vi "DockerTools - Get container list.vi"(8 "error in":errorcluster) -> (0 "error out":errorcluster, 2 "Container list":string[][](array[string]), 3 "Standard output":string)   [LabVIEW 2017]
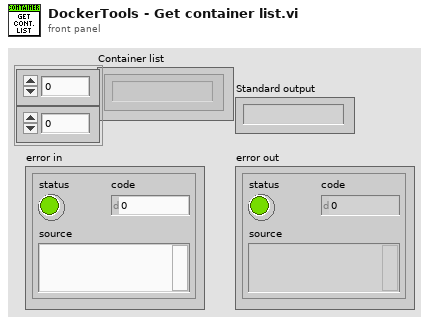
[diagram p1: front panel]
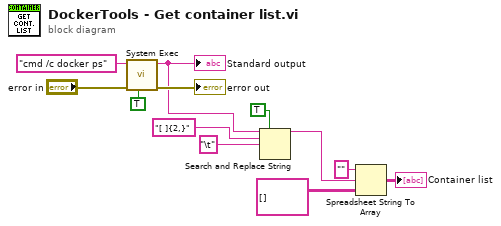
[diagram p0: block diagram]
diagram:
  n1 = call <vilib>:"System Exec.vi"("run minimized? (F)"=TRUE, "error in (no error)"="error in", "command line"="cmd /c docker ps") -> ("error out"=→"error out":errorcluster, "standard output"=w2:string)  [unwired: 5 in, 2 out]
  "Standard output" <- w2
  n2 = Search and Replace String(replace all?=TRUE ("replace all? (F)"), input string=w2, search string="[ ]{2,}", replace string="\t" ("replace string (\"\")")) -> (result string=w4:string)  [unwired: 4 in, 3 out]
  n3 = Spreadsheet String To Array(format string="", spreadsheet string=w4, array type (2D Dbl)=string[][] []) -> (array=→"Container list":string[][])  [unwired: 1 in]
